vi "CalculateThickness.vi"(10 "Speed Of Sound":dbl, 11 "AScan+Peaks":cluster{"timebase":dbl[], "data":u16[]}[](array[cluster])) -> (3 "Thickness [mm]":dbl[](array[numeric]))   [LabVIEW 2026]
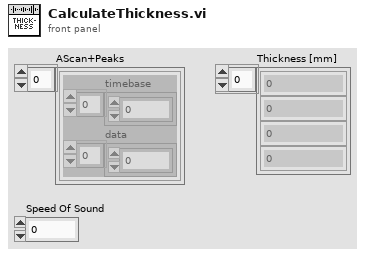
[diagram p1: front panel]
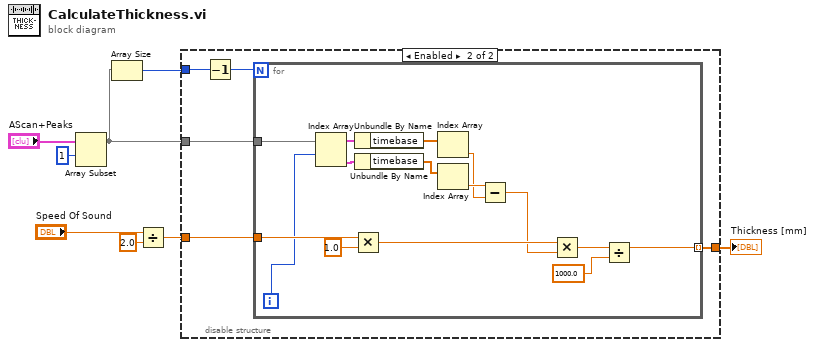
[diagram p0: block diagram]
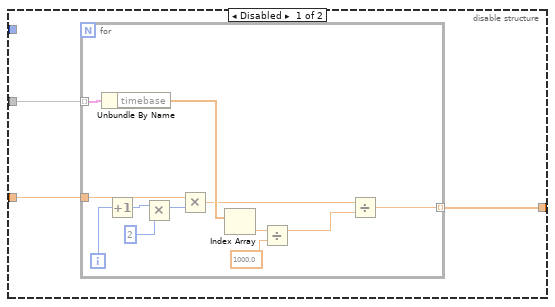
[diagram p2: hidden frame]
diagram:
  n1 = Array Subset(array="AScan+Peaks", index=1) -> (w4:cluster{"timebase":dbl[], "data":u16[]}[])  [unwired: 1 in]
  n2 = Array Size(array=w4) -> (size(s)=w3:i32)
  n3 = Divide(x="Speed Of Sound", y=2.0) -> (x/y=w1:dbl)
  n4 = disable-structure shown="Enabled" {
    disable-tunnel: w1 -> [w11 w28]
    disable-tunnel: [w10 w27] -> w7
    disable-tunnel: w4 -> [w9 w26]
    disable-tunnel: w3 -> [_ w25]
    frame Disabled {
      n5 = for {
        tunnel: w9 -> [w23] mode=indexing
        tunnel: w11 -> [w21]
        tunnel: [w19] -> w10 mode=indexing
        i -> [w15]
        n6 = Unbundle By Name(w23) -> ("timebase"=w22:dbl[])
        n7 = Increment(x=w15) -> (x+1=w14:i32)
        n8 = Multiply(x=w14, y=2 ("x")) -> (x*y=w13:i32)
        n9 = Multiply(x=w21, y=w13) -> (x*y=w16:dbl)
        n10 = Index Array(array=w22) -> (element=w20:dbl)  [unwired: 1 in]
        n11 = Divide(x=w20, y=1000.0) -> (x/y=w18:dbl)
        n12 = Divide(x=w16, y=w18) -> (x/y=w19:dbl)
      }
    }
    frame Enabled {
      n13 = Decrement(x=w25) -> (x-1=w24:i32)
      n14 = for {
        N: w24 -> [_]
        tunnel: w26 -> [w43]
        tunnel: w28 -> [w41]
        tunnel: [w30] -> w27 mode=indexing
        i -> [w32]
        n15 = Index Array(array=w43, index #1=w32) -> (element #1=w38:cluster{"timebase":dbl[], "data":u16[]}, element #2=w37:cluster{"timebase":dbl[], "data":u16[]})  [unwired: 1 in]
        n16 = Multiply(x=w41, y=1.0) -> (x*y=w39:dbl)
        n17 = Unbundle By Name(w38) -> ("timebase"=w42:dbl[])
        n18 = Unbundle By Name(w37) -> ("timebase"=w36:dbl[])
        n19 = Index Array(array=w42) -> (element=w34:dbl)  [unwired: 1 in]
        n20 = Index Array(array=w36) -> (element=w35:dbl)  [unwired: 1 in]
        n21 = Subtract(x=w35, y=w34) -> (x-y=w31:dbl)
        n22 = Multiply(x=w39, y=w31) -> (x*y=w40:dbl)
        n23 = Divide(x=w40, y=1000.0) -> (x/y=w30:dbl)
      }
    }
  }
  "Thickness [mm]" <- w7
